vi "Generate DO waveform.vi"(11 "Status":T1 {"Setting"."X Pos." scale=-5.0..5.0; "Setting"."Y Pos." scale=-5.0..5.0}) -> (0 "low time":dbl, 1 "High Time":dbl, 2 "大小":i32, 3 "Digital Signal":digitalwaveform(graph))   [LabVIEW 2013]
uses:
  init & communication/init-status.ctl
  init & communication/Setting.ctl
  init & communication/event-package.ctl
  init & communication/Event1.ctl
  init & communication/data-package.ctl
  init & communication/Event.ctl
  <vilib>/Waveform/DWDTOps.llb/Digital Pattern Generator (Single Value).vi
  <vilib>/Waveform/DWDTOps.llb/DWDT Append Digital Samples.vi
  <vilib>/Waveform/DWDTOps.llb/DWDT Digital Size.vi
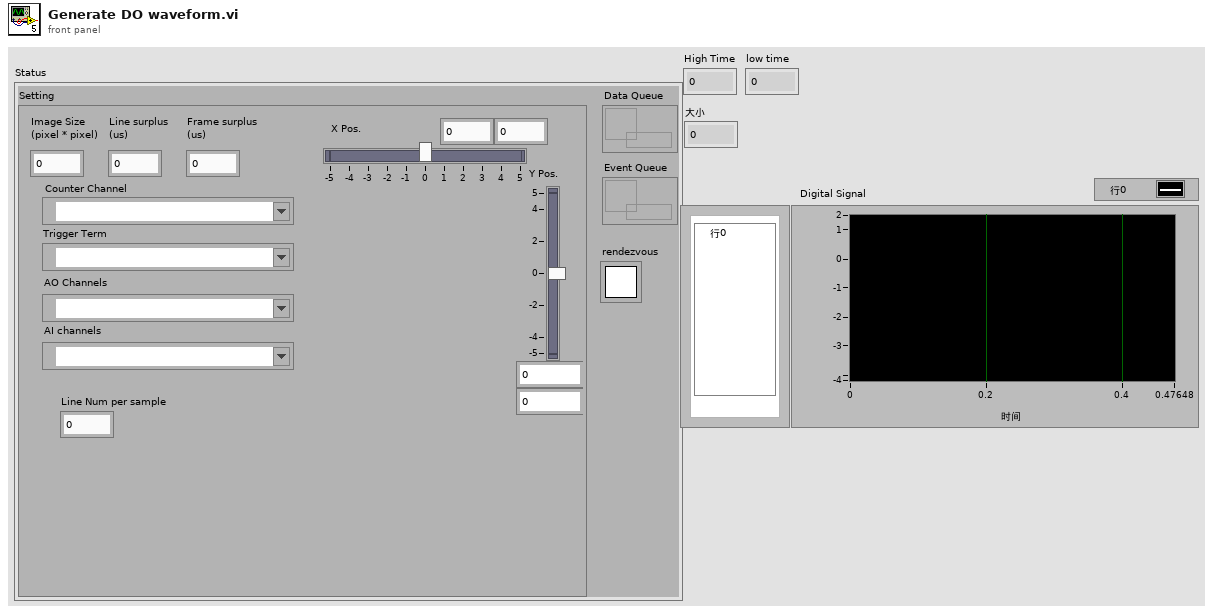
[diagram p1: front panel]
types:
  T1 = typedef "init-status.ctl" = cluster{"Setting":T2, "Event Queue":refnum<queue>, "Data Queue":refnum<queue>, "rendezvous":T3}
  T2 = typedef "Setting.ctl" = cluster{"Image Size\n(pixel * pixel)":i32, "Counter Channel":tag, "Trigger Term":tag, "AO Channels":tag, "Y Pos.":cluster{dbl, dbl}, "X Pos.":cluster{dbl, dbl}, "Line surplus\n(us)":i32, "Frame surplus\n(us)":i32, "AI channels":tag, "Line Num per sample":i32}
  T3 = typedef "Rendezvous RefNum" = refnum<k1>
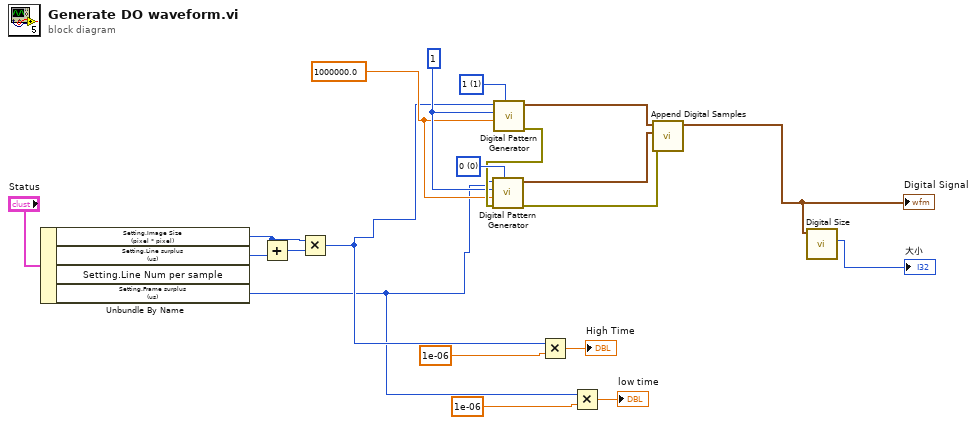
[diagram p0: block diagram]
diagram:
  w10 = 1000000.0 ("sample rate")
  w11 = u32 1 ("number of signals")
  w15 = u8 0 items=["0", "1", "Z", "L", "H", "X", "T", "V"] ("value")
  w16 = u8 1 items=["0", "1", "Z", "L", "H", "X", "T", "V"] ("value")
  n1 = Unbundle By Name("Status") -> ("Setting.Image Size\n(pixel * pixel)"=w17:i32, "Setting.Line surplus\n(us)"=w19:i32, "Setting.Frame surplus\n(us)"=w3:i32)  [unwired: 1 out]
  n2 = Add(x=w17, y=w19) -> (x+y=w18:i32)
  n3 = Multiply(x=w17, y=w18) -> (x*y=w6:i32)
  n4 = call-poly <vilib>:"Digital Pattern Generator.vi"("value"=w16, "sample rate"=w10, "number of signals"=w11, "number of samples"=w6) -> ("error out"=w13:errorcluster, "digital waveform"=w9:digitalwaveform)  [unwired: 6 in]
  n5 = call-poly <vilib>:"Digital Pattern Generator.vi"("value"=w15, "error in (no error)"=w13, "sample rate"=w10, "number of signals"=w11, "number of samples"=w3) -> ("error out"=w12:errorcluster, "digital waveform"=w14:digitalwaveform)  [unwired: 5 in]
  n6 = Multiply(x=w6, y=1e-06) -> (x*y=→"High Time":dbl)
  n7 = Multiply(x=w3, y=1e-06) -> (x*y=→"low time":dbl)
  n8 = call-poly <vilib>:"Append Digital Samples.vi"("error in (no error)"=w12, "digital waveform B"=w14, "digital waveform A"=w9) -> ("digital waveform out"=w7:digitalwaveform)  [unwired: 7 in, 1 out]
  "Digital Signal" <- w7
  n9 = call-poly <vilib>:"Digital Size.vi"("digital waveform in"=w7) -> ("number of samples"=→"大小":i32)  [unwired: 7 in, 3 out]
